vi "Store Active Observer.vi"(8 "error in (no error)":errorcluster, 10 "Observer In":refnum<class "Observer.lvclass">, 11 "Vessel in":refnum<class "Vessel.lvclass">) -> (0 "error out":errorcluster, 3 "Vessel out":refnum<class "Vessel.lvclass">)   [LabVIEW 2014, in "Vessel.lvclass"]
uses:
  Vessel.lvclass
  Observer/Observer.lvclass
  Vessel.lvclass/Vessel.ctl
  Supervisor/Supervisor.lvclass
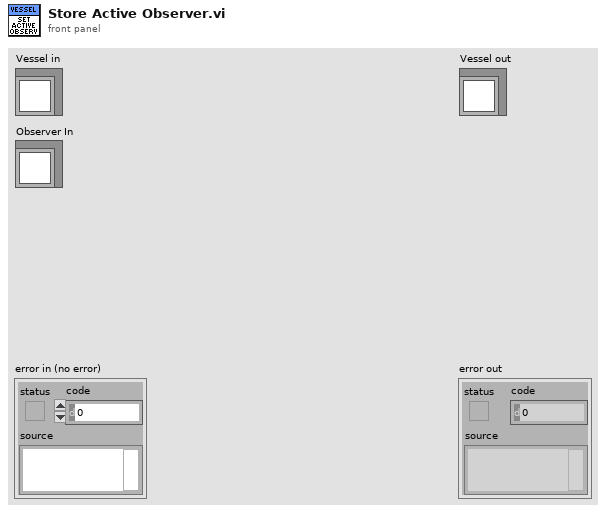
[diagram p1: front panel]
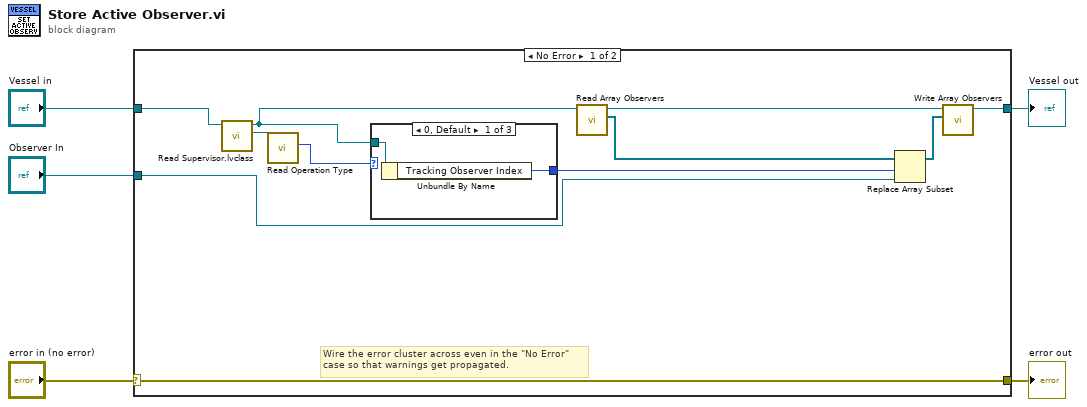
[diagram p0: block diagram]
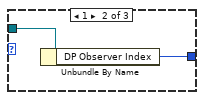
[diagram p2: hidden frame]
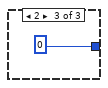
[diagram p3: hidden frame]
diagram:
  n1 = case shown="No Error" "error in (no error)" {
    selector: "error in (no error)" -> [w16 w23]
    tunnel: [w16 w23] -> w4
    tunnel: [w10 w22] -> w2
    tunnel: "Vessel in" -> [w15 w22]
    tunnel: "Observer In" -> [w7 _]
    frame No Error {
      # "Wire the error cluster across even in the \"No Error\"\ncase so that warnings get propagated."
      n2 = call "Read Supervisor.lvclass.vi"("Vessel in"=w15) -> ("Supervisor.lvclass"=w14:refnum<class "Supervisor.lvclass">, "Vessel out"=w11:refnum<class "Vessel.lvclass">)  [unwired: 8 in, 1 out]
      n3 = call-dynamic "Read Operation Type.vi"("Supervisor in"=w14) -> ("Operation Type"=w13:u16)  [unwired: 8 in, 2 out]
      n4 = case shown="0, Default" w13 {
        tunnel: w11 -> [w18 w20 _]
        tunnel: [w17 w19 0] -> w6
        frame 0, Default {
          n5 = Unbundle By Name(w18) -> ("Tracking Observer Index"=w17:i32)
        }
        frame 1 {
          n6 = Unbundle By Name(w20) -> ("DP Observer Index"=w19:i32)
        }
        frame 2 {
        }
      }
      n7 = call-dynamic "Read Array Observers.vi"("Vessel in"=w11) -> ("Array Observers"=w12:refnum<class "Observer.lvclass">[], "Vessel out"=w8:refnum<class "Vessel.lvclass">)  [unwired: 8 in, 1 out]
      n8 = Replace Array Subset(array=w12, new element=w7, index=w6) -> (w9:refnum<class "Observer.lvclass">[])
      n9 = call-dynamic "Write Array Observers.vi"("Array Observers"=w9, "Vessel in"=w8) -> ("Vessel out"=w10:refnum<class "Vessel.lvclass">)  [unwired: 8 in, 1 out]
    }
    frame Error {
    }
  }
  "error out" <- w4
  "Vessel out" <- w2
